vi "E710_InitialisationOfWaveScan.vi"(0 "amplitude":dbl, 7 "Fast Axis":string="1", 8 "Slow Axis Steps":dbl, 11 "error in":errorcluster, 12 "FastAxisStepsize":dbl, 13 "kineticexposure":dbl) -> (4 "scan time for 1 line/sec":dbl=200.0 format="%.3g", 6 "scan time for 1 area/sec 2":dbl=200.0 format="%.3g", 15 "error out 2":errorcluster)   [LabVIEW 2011]
doc: "This VI initializes and configures the E-710 to perform a XY scan."
uses:
  Utilities/controls/ctlSeqFNs_PI_SysNr.ctl
  Variables/GlobalSetNumberOfDigits_Scanners.vi
  Variables/GlobalCameraDebugTemperature.vi
panel:
  out "Active High":u32[](array[numeric]) format="%.0x"
  out "Aktibe High":dbl[](array[numeric]) format="%.6f"
  out "Trigger pulse length":u32[](array[numeric]) format="%.0x"
  out "Trigger pulse length":dbl[](array[numeric]) format="%.6f"
  out "Wavegenerator Cycles":u32[](array[numeric]) format="%.0x"
  out "Wavegenerator Cycles":dbl[](array[numeric]) format="%.6f"
  # "E-710 Wavescan Initialization"
  # "This VI initializes and configures the E-710 to perform a XY raster scan. Scan motion in X axis can be uni-\nor bidirectional. Triggerline 1 fires on waveform start."
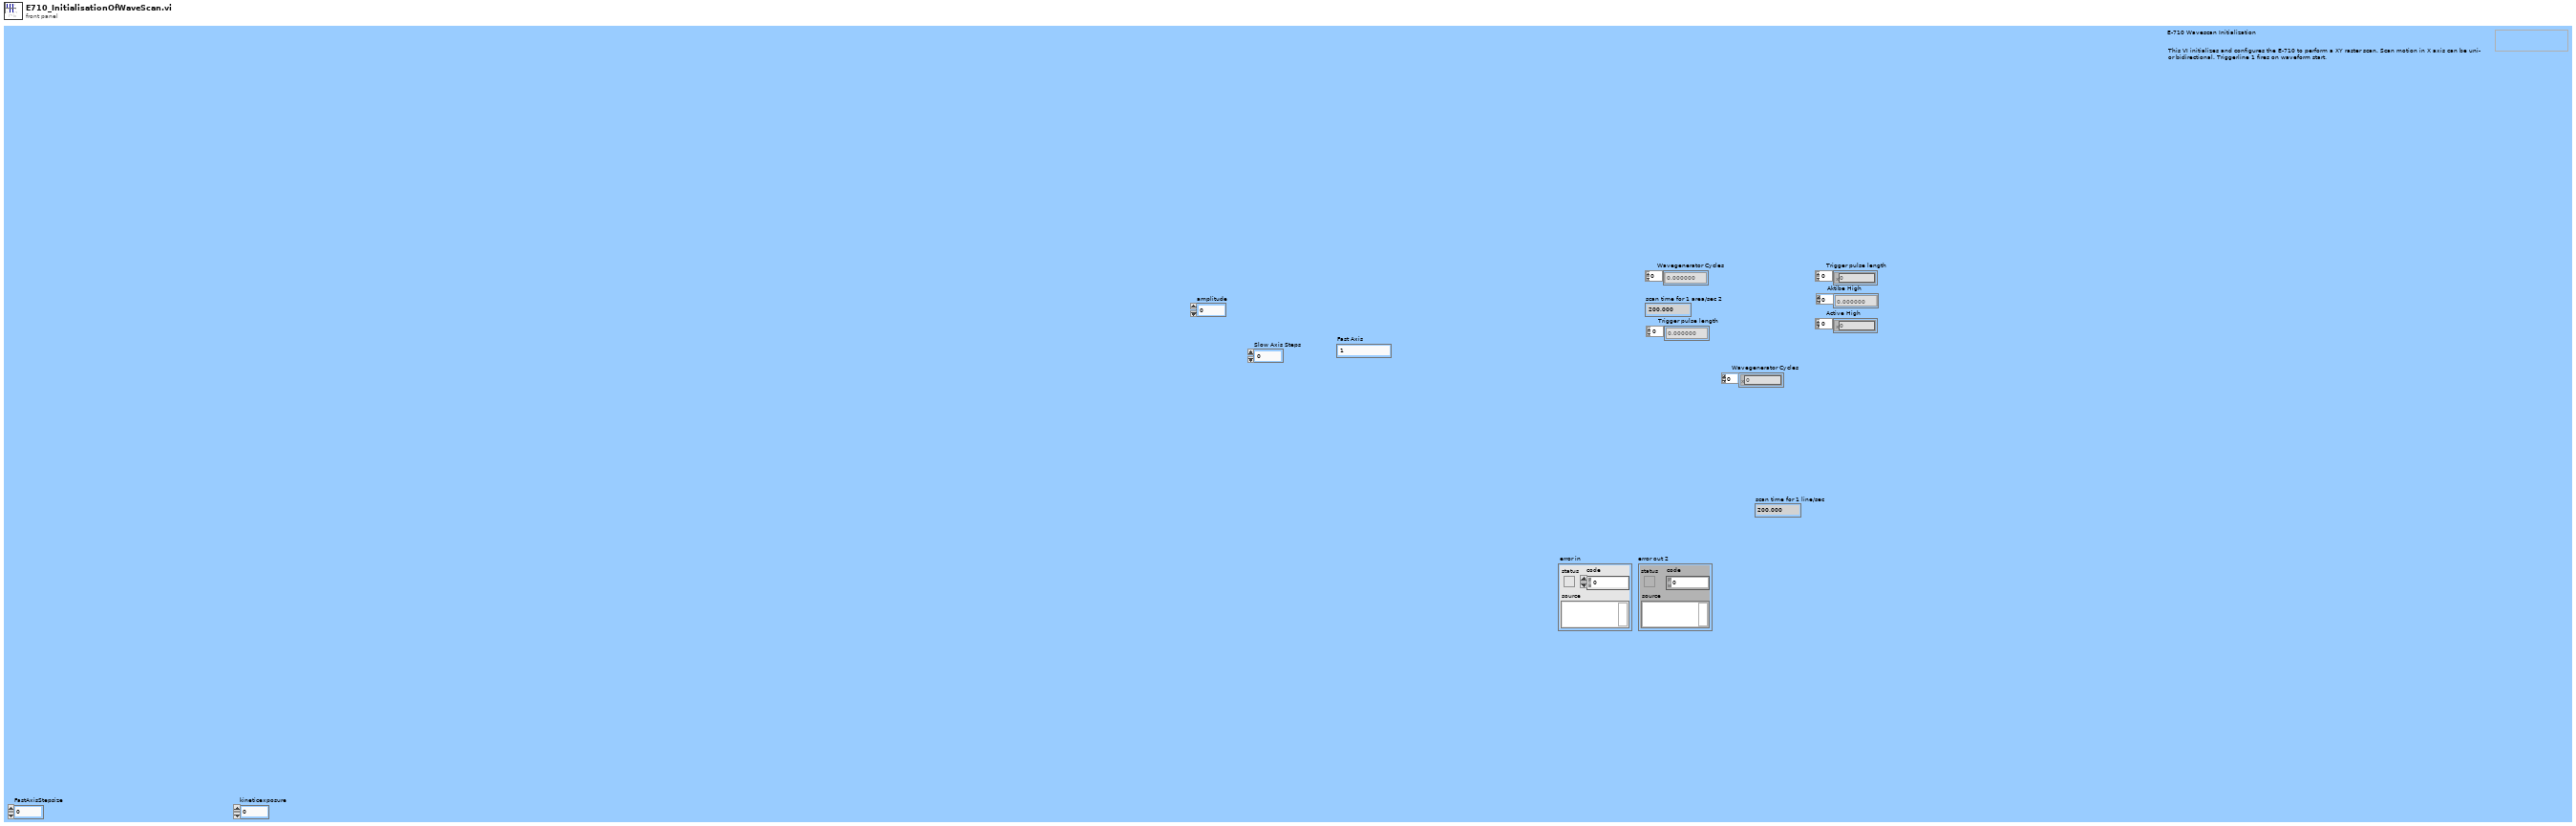
[diagram p1: front panel]
types:
  T1 = typedef "ctlSeqFNs_PI_SysNr.ctl" = enum16{"Zero", "E517", "E710"}
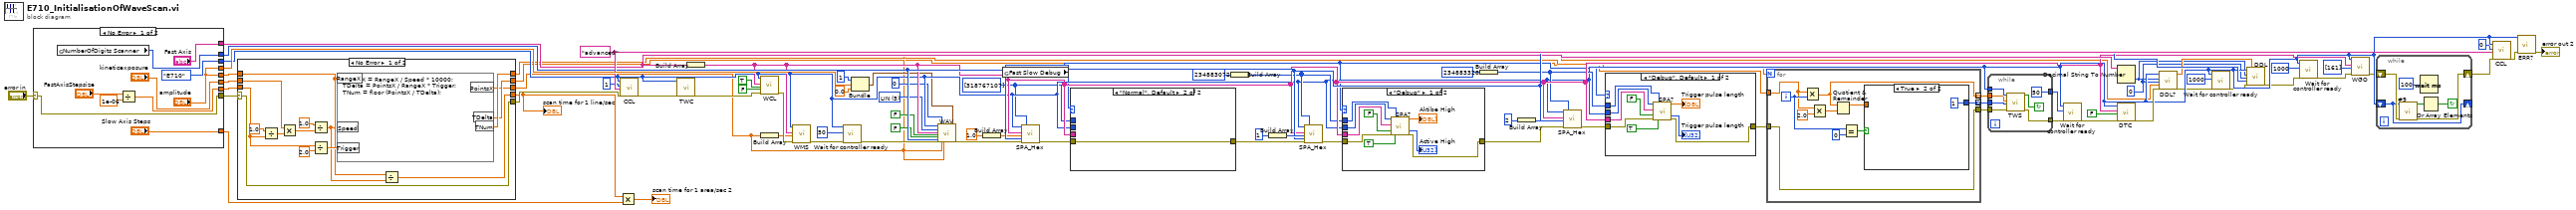
[diagram p0: block diagram]
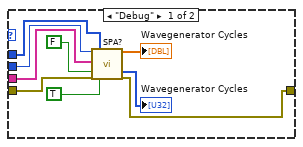
[diagram p3: hidden frame]
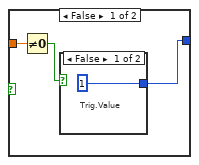
[diagram p4: hidden frame]
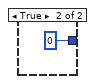
[diagram p5: hidden frame]
diagram:
  w15 = 0 ("Offset")
  w29 = u32[] [318767107] ("Parameter number (hex)")
  w46 = u16 5 items=["SIN", "POL", "TAN", "PNT", "SIN_P", "LIN", "RAMP"] ("Waveform")
  w70 = "advanced" ("Password")
  n1 = case shown="No Error" "error in" {
    selector: "error in" -> [w83 w88]
    tunnel: ["amplitude" _] -> w73
    tunnel: ["Fast Axis" _] -> w57
    tunnel: [ctlSeqFNs_PI_SysNr."E710" ("STATE") _] -> w50
    tunnel: [w85 _] -> w63
    tunnel: ["Slow Axis Steps" _] -> w62
    tunnel: [w83 w88] -> w26
    tunnel: ["kineticexposure" _] -> w28
    tunnel: ["amplitude" _] -> w24
    tunnel: [w79 _] -> w27
    frame No Error {
      n2 = global read "GlobalSetNumberOfDigits_Scanners.vi" "NumberOfDigits Scanner"() -> (w85:i32)
      n3 = Divide(x="FastAxisStepsize", y=1e-06) -> (x/y=w79:dbl)
    }
    frame Error {
    }
  }
  n4 = case shown="No Error" w26 {
    selector: w26 -> [w100 _]
    tunnel: [w103 _] -> w47
    tunnel: [w102 _] -> w1
    tunnel: w28 -> [w96 _]
    tunnel: w24 -> [w90 _]
    tunnel: w27 -> [w93 _]
    tunnel: [w101 _] -> w2
    tunnel: [w100 _] -> w25
    tunnel: [w99 _] -> w23
    frame No Error {
      n5 = Divide(x=1.0, y=w93) -> (x/y=w97:dbl)
      n6 = Multiply(x=w96, y=w97) -> (x*y=w95:dbl)
      n7 = Divide(x=1.0, y=w95) -> (x/y=w89:dbl)
      n8 = Divide(x=w93, y=2.0) -> (x/y=w91:dbl)
      n9 = formula code="PointsX = RangeX / Speed * 10000;\nTDelta = PointsX / RangeX * Trigger;\nTNum = floor (PointsX / TDelta);"("RangeX"=w90, "Speed"=w89, "Trigger"=w91) -> ("PointsX"=w101:dbl, "TDelta"=w102:dbl, "TNum"=w103:dbl)
      n10 = Divide(x=w90, y=w89) -> (x/y=w99:dbl)
    }
    frame Error {
    }
  }
  "scan time for 1 line/sec" <- w23
  n11 = Multiply(x=w23, y=w62) -> (x*y=→"scan time for 1 area/sec 2":dbl)
  n12 = call "CCL.vi"("System no."=w50, "Command level"=1, "Password"=w70, "error in"=w25) -> ("error out"=w72:errorcluster)  [unwired: 14 in, 1 out]
  n13 = call "TWC.vi"("System no."=w50, "error in"=w72) -> ("error out"=w65:errorcluster)  [unwired: 17 in]
  n14 = Build Array(w57) -> (w53:string[])
  n15 = call "WCL.vi"("System no."=w50, "WCL axes"=w53, "All axes?"=TRUE, "Axis identifier?"=FALSE, "error in"=w65) -> ("error out"=w37:errorcluster)  [unwired: 14 in]
  n16 = Build Array(w2) -> (w35:dbl[])
  n17 = call "WMS.vi"("System no."=w50, "Axes to set"=w53, "Wave storage max."=w35, "error in"=w37) -> ("error out"=w39:errorcluster)  [unwired: 14 in, 1 out]
  n18 = call "Wait for controller ready.vi"("System no."=w50, "Polling time, ms"=50, "error in"=w39) -> ("error out"=w36:errorcluster)  [unwired: 15 in, 1 out]
  n19 = Bundle("y"=1, "amplitude"=w73, "O"=0.0) -> (w44:cluster{"y":i32, "amplitude":dbl, "O":dbl})  [unwired: 1 in]
  n20 = call "WAV.vi"("System no."=w50, "Waveform"=w46, "Affected axes"=w53, "Append? (&)"=FALSE, "Add? (+)"=FALSE, "No.of digits"=w63, "error in"=w36, "Xo"=0, "N"=w2, "Segment length"=w2, "LIN Parameters"=w44) -> ("error out"=w9:errorcluster)  [unwired: 15 in, 1 out]
  n21 = Build Array(1.0 ("element")) -> (w34:dbl[])
  n22 = global read "GlobalCameraDebugTemperature.vi" "Fast Slow Debug"() -> (w48:enum32{"Normal", "Debug"})
  n23 = call "SPA_Hex.vi"("System no."=w50, "Designator to set"=w53, "Parameter value"=w34, "No.of digits"=w63, "error in"=w9, "Parameter number (hex)"=w29) -> ("error out"=w30:errorcluster)  [unwired: 12 in, 1 out]
  n24 = case shown="\"Normal\", Default" w48 {
    tunnel: w30 -> [w110 w113]
    tunnel: [w109 w113] -> w64
    tunnel: w50 -> [w108 _]
    tunnel: w53 -> [w107 _]
    tunnel: w29 -> [w106 _]
    frame "Debug" {
      n25 = call "SPA?.vi"("System no."=w108, "Axes to query"=w107, "Without axes?"=FALSE, "error in"=w110, "Parameter no. (hex)"=w106, "Parameter no. format \n(Decimal: FALSE)"=TRUE ("Parameter no. format \n(Decimal: FALSE)")) -> ("Parameter value"=→"Wavegenerator Cycles":dbl[], "Parameter no. (hex) out"=→"Wavegenerator Cycles":u32[], "error out"=w109:errorcluster)  [unwired: 8 in, 3 out]
    }
    frame "Normal", Default {
    }
  }
  n26 = Build Array(u32 234883072 ("Numeric")) -> (w52:u32[])
  n27 = Build Array(i16 1 ("element")) -> (w77:i16[])
  n28 = call "SPA_Hex.vi"("System no."=w50, "Designator to set"=w53, "Parameter value"=w77, "No.of digits"=w63, "error in"=w64, "Parameter number (hex)"=w52) -> ("error out"=w56:errorcluster)  [unwired: 12 in, 1 out]
  n29 = case shown="\"Debug\"" w48 {
    tunnel: w56 -> [w122 w123]
    tunnel: [w121 w123] -> w55
    tunnel: w53 -> [w120 _]
    tunnel: w52 -> [w119 _]
    tunnel: w50 -> [w114 _]
    frame "Debug" {
      n30 = call "SPA?.vi"("System no."=w114, "Axes to query"=w120, "Without axes?"=FALSE, "error in"=w122, "Parameter no. (hex)"=w119, "Parameter no. format \n(Decimal: FALSE)"=TRUE ("Parameter no. format \n(Decimal: FALSE)")) -> ("Parameter value"=→"Aktibe High":dbl[], "Parameter no. (hex) out"=→"Active High":u32[], "error out"=w121:errorcluster)  [unwired: 8 in, 3 out]
    }
    frame "Normal", Default {
    }
  }
  n31 = Build Array(234883328 ("Numeric")) -> (w51:i32[])
  n32 = Build Array(2 ("element")) -> (w76:i32[])
  n33 = call "SPA_Hex.vi"("System no."=w50, "Designator to set"=w53, "Parameter value"=w76, "No.of digits"=w63, "error in"=w55, "Parameter number (hex)"=w51) -> ("error out"=w54:errorcluster)  [unwired: 12 in, 1 out]
  n34 = case shown="\"Debug\", Default" w48 {
    tunnel: w54 -> [w132 w133]
    tunnel: [w131 w133] -> w4
    tunnel: w53 -> [w130 _]
    tunnel: w51 -> [w129 _]
    tunnel: w50 -> [w125 _]
    frame "Debug", Default {
      n35 = call "SPA?.vi"("System no."=w125, "Axes to query"=w130, "Without axes?"=FALSE, "error in"=w132, "Parameter no. (hex)"=w129, "Parameter no. format \n(Decimal: FALSE)"=TRUE ("Parameter no. format \n(Decimal: FALSE)")) -> ("Parameter value"=→"Trigger pulse length":dbl[], "Parameter no. (hex) out"=→"Trigger pulse length":u32[], "error out"=w131:errorcluster)  [unwired: 8 in, 3 out]
    }
    frame "Normal" {
    }
  }
  n36 = for {
    N: w47 -> [_]
    tunnel: w1 -> [w134]
    tunnel: [w137] -> w11 mode=indexing
    tunnel: [w143] -> w10 mode=indexing
    tunnel: w4 -> [w138]
    tunnel: [w138] -> w3
    i -> [w141]
    n37 = Multiply(x=w134, y=w141) -> (x*y=w137:dbl)
    n38 = Multiply(x=w134, y=2.0) -> (x*y=w136:dbl)
    n39 = Quotient & Remainder(x=w137, y=w136) -> (x-y*floor(x/y)=w142:dbl)  [unwired: 1 out]
    n40 = Equal?(x=w141, y=0) -> (x = y?=w139:bool)
    n41 = case shown="True" w139 {
      tunnel: [w146 1] -> w143
      tunnel: w142 -> [w145 _]
      frame False {
        n42 = Not Equal To 0?(x=w145) -> (x != 0?=w144:bool)
        n43 = case shown="False" w144 {
          tunnel: [1 0] -> w146
          frame False {
            # "Trig.Value"
          }
          frame True {
          }
        }
      }
      frame True {
      }
    }
  }
  n44 = while {
    tunnel: [50 ("Polling time, ms")] -> w71
    tunnel: [w155] -> w49
    tunnel: w3 -> [w154]
    tunnel: w50 -> [w153]
    tunnel: w11 -> [w151]
    tunnel: w10 -> [w150]
    stop <- w152 continue-if-true
    n45 = call "TWS.vi"("System no."=w153, "Wavepoint"=w151, "Trigger value"=w150, "error in"=w154) -> ("Controller error"=w152:bool, "error out"=w155:errorcluster)  [unwired: 14 in]
  }
  n46 = call "Wait for controller ready.vi"("System no."=w50, "Polling time, ms"=w71, "error in"=w49) -> ("error out"=w69:errorcluster)  [unwired: 15 in, 1 out]
  n47 = Decimal String To Number(string=w57) -> (number=w17:i32)  [unwired: 2 in, 1 out]
  n48 = call "DTC.vi"("System no."=w50, "DDL table"=w53, "All tables?"=FALSE, "error in"=w69) -> ("error out"=w67:errorcluster)  [unwired: 15 in]
  n49 = call "DDL?.vi"("System no."=w50, "Table no."=w17, "Offset"=w15, "N"=w2, "error in"=w67) -> ("Values"=w21:dbl[], "error out"=w20:errorcluster)  [unwired: 13 in]
  n50 = call "Wait for controller ready.vi"("System no."=w50, "Polling time, ms"=1000, "error in"=w20) -> ("error out"=w19:errorcluster)  [unwired: 15 in, 1 out]
  n51 = call "DDL.vi"("System no."=w50, "Table no."=w17, "Offset"=w15, "No.of digits"=w63, "error in"=w19, "Values"=w21) -> ("error out"=w18:errorcluster)  [unwired: 13 in]
  n52 = call "Wait for controller ready.vi"("System no."=w50, "Polling time, ms"=1000, "error in"=w18) -> ("error out"=w14:errorcluster)  [unwired: 15 in, 1 out]
  n53 = call "WGO.vi"("System no."=w50, "Affected axes"=w53, "WGO Parameter"=i32[] [161], "error in"=w14) -> ("error out"=w12:errorcluster)  [unwired: 14 in, 1 out]
  n54 = while {
    shift-right: [w161] -> w60
    shift-left: w12 -> [w162]
    shift-right: [w159] -> _
    shift-left: w50 -> [w159]
    stop <- w157 continue-if-true
    n55 = call "#9.vi"("System no."=w159, "error in"=w162) -> ("WG running?"=w158:bool[], "error out"=w161:errorcluster)  [unwired: 16 in]
    n56 = Wait (ms)(milliseconds to wait=u32 100) -> ()  [unwired: 1 out]
    n57 = Or Array Elements(Boolean array=w158) -> (logical OR=w157:bool)
  }
  n58 = call "CCL.vi"("System no."=w50, "Command level"=0, "Password"=w70, "error in"=w60) -> ("error out"=w75:errorcluster)  [unwired: 14 in, 1 out]
  n59 = call "ERR?.vi"("System no."=w50, "error in"=w75) -> ("error out"=→"error out 2":errorcluster)  [unwired: 16 in, 1 out]
